vi "Experiment-2_4526.vi"() -> ()   [LabVIEW 2021]
uses:
  <vilib>/httpClient/LabVIEWHTTPClient.lvlib
panel:
  out "error out":errorcluster
  out "body - Output from thingspeak channel":string
  out "headers":string
  in  "stop":bool
  in  "error in (no error)":errorcluster
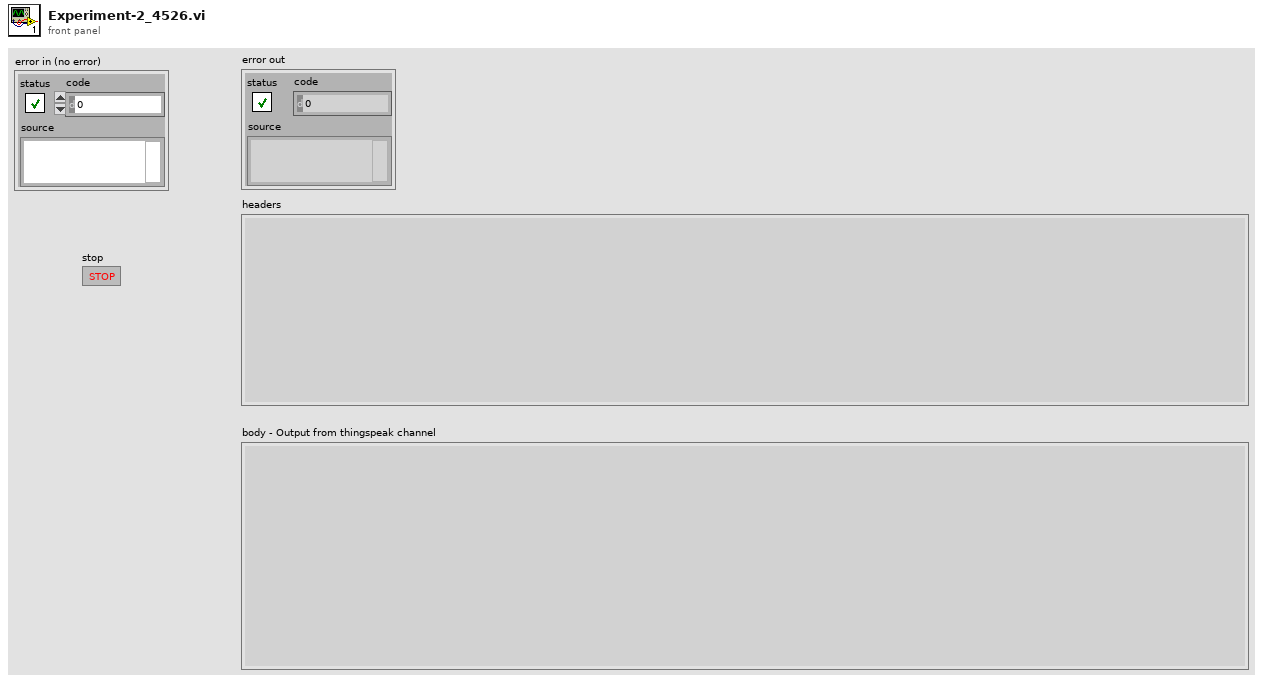
[diagram p1: front panel]
types:
  T1 = typedef "LabVIEWHTTPClient.lvlib/ClientHandle.ctl" = refnum<k1>
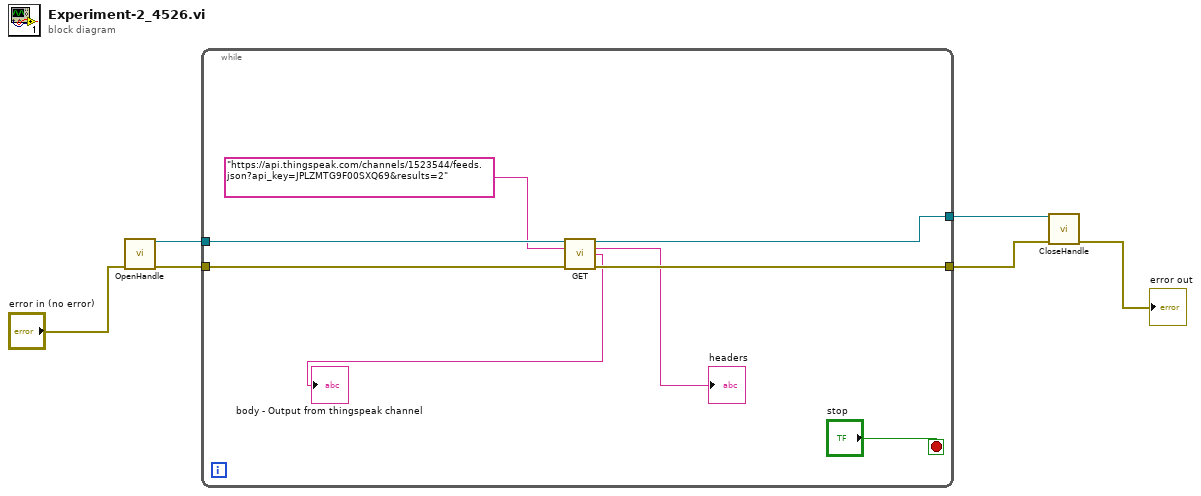
[diagram p0: block diagram]
diagram:
  n1 = call <vilib>:"OpenHandle.vi"("error in (no error)"="error in (no error)") -> ("client handle out"=w6:T1, "error out"=w3:errorcluster)  [unwired: 13 in]
  n2 = while {
    tunnel: w6 -> [w14]
    tunnel: [w13] -> w5
    tunnel: w3 -> [w12]
    tunnel: [w11] -> w2
    stop <- "stop" stop-if-true
    n3 = call <vilib>:"GET.vi"("client handle"=w14, "url"="https://api.thingspeak.com/channels/1523544/feeds.json?api_key=JPLZMTG9F00SXQ69&results=2", "error in (no error)"=w12) -> ("client handle out"=w13:T1, "headers"=→"headers":string, "body"=→"body - Output from thingspeak channel":string, "error out"=w11:errorcluster)  [unwired: 9 in]
  }
  n4 = call <vilib>:"CloseHandle.vi"("client handle"=w5, "error in (no error)"=w2) -> ("error out"=→"error out":errorcluster)  [unwired: 13 in]
